vi "VG_DCIRmin.vi"() -> ()   [LabVIEW 2020]
panel:
  out "DCIRmin":dbl
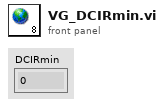
[diagram p1: front panel]
diagram:
